vi "OnShot.vi"() -> ()   [LabVIEW 2024]
uses:
  <vilib>/DAQmx/read.llb/DAQmx Read (Analog DBL 1Chan 1Samp).vi
  <vilib>/DAQmx/create/channels.llb/DAQmx Create Channel (AI-Voltage-Basic).vi
  <vilib>/DAQmx/miscellaneous.llb/DAQmx Fill In Error Info.vi
panel:
  in  "input terminal configuration":i32(ring)=-1 items=["Default"=-1, "RSE"=10083, "NRSE"=10078, "Differential"=10106, "Pseudodifferential"=12529]
  out "data":dbl format="%0.2f"
  in  "physical channels":tag
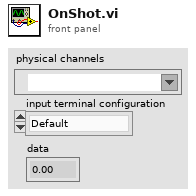
[diagram p1: front panel]
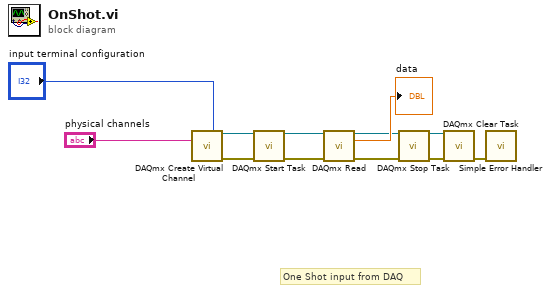
[diagram p0: block diagram]
diagram:
  # "One Shot input from DAQ"
  n1 = call-poly <vilib>:"DAQmx Create Virtual Channel.vi"("input terminal configuration"="input terminal configuration", "physical channels"="physical channels") -> ("task out"=w11:refnum<k21>, "error out"=w10:errorcluster)  [unwired: 12 in]
  n2 = call <vilib>:"DAQmx Start Task.vi"("task/channels in"=w11, "error in"=w10) -> ("task out"=w9:refnum<k21>, "error out"=w8:errorcluster)  [unwired: 12 in]
  n3 = call-poly <vilib>:"DAQmx Read.vi"("task/channels in"=w9, "error in"=w8) -> ("task out"=w6:refnum<k21>, "data"=→"data":dbl, "error out"=w4:errorcluster)  [unwired: 11 in]
  n4 = call <vilib>:"DAQmx Stop Task.vi"("task/channels in"=w6, "error in"=w4) -> ("task out"=w5:refnum<k21>, "error out"=w3:errorcluster)  [unwired: 12 in]
  n5 = call <vilib>:"DAQmx Clear Task.vi"("task in"=w5, "error in"=w3) -> ("error out"=w1:errorcluster)  [unwired: 13 in]
  n6 = call <vilib>:"Simple Error Handler.vi"("error in (no error)"=w1) -> ()  [unwired: 4 in, 5 out]
